vi "SDT_MeasureBlockToString.vi"(11 "MeasureInfo":T1={"mod_ser_no"="3F0024\u0000\u0000\u0000\u0000\u0000\u0000\u0000\u0000\u0000\u0000", "MeasureInfo_PartB"={"meas_mode"=13, "cfd_ll"=-29.411764, "cfd_lh"=5.019608, "cfd_zc"=12.850393, "cfd_hf"=5.0, "syn_zc"=-5.2913384, "syn_fd"=1, "syn_hf"=4.0, "tac_r"=5.0033574e-08, "tac_g"=3, "tac_of"=7.45098, "tac_ll"=5.098039, "tac_lh"=95.29412, "adc_re"=4096, "eal_de"=0, "ncx"=1, "ncy"=1, "page"=1, "col_t"=20.0, "rep_t"=20.0, "stopt"=0, "overfl"=78, "use_motor"=0, "steps"=1, "offset"=0.0, "dither"=128, "incr"=1, "mem_bank"=0, "mod_type1"=3722795091, "mod_type2"=0, "syn_th"=-50.980392, "dead_time_comp"=0, "polarity_l"=1, "polarity_f"=1, "polarity_p"=1, "linediv"=0, "accumulate"=0, "flbck_y"=1, "flbck_x"=1, "bord_u"=0, "bord_l"=0, "pix_time"=2e-07, "pix_clk"=1, "trigger"=16, "scan_x"=512, "scan_y"=512, "scan_rx"=1, "scan_ry"=1, "fifo_typ"=0, "epx_div"=1, "mod_type_code"=150, "mod_fpga_ver"=514, "overflow_corr_factor"=0.0, "adc_zoom"=0, "cycles"=1}, "MeasStopInfo"={"status"=824, "flags"=33199, "stop_time"=377.24805, "cur_step"=1, "cur_cycle"=1, "cur_page"=1, "min_sync_rate"=12634368.0, "min_cfd_rate"=1056.0, "min_tac_rate"=1056.0, "min_adc_rate"=70432.0, "max_sync_rate"=40678656.0, "max_cfd_rate"=769936.0, "max_tac_rate"=581984.0, "max_adc_rate"=565856.0, "reserved1"=0, "reserved2"=0.0}, "MeasFCSInfo"={"chan"=1, "fcs_decay_calc"=32, "mt_resol"=250, "cortime"=1.0, "calc_photons"=164220395, "fcs_points"=0, "end_time"=377.2369, "overruns"=0, "fcs_type"=32801, "cross_chan"=8, "mod"=0, "cross_mod"=0, "cross_mt_resol"=250}, "MeasureInfo_PartE"={"image_x"=512, "image_Y"=512, "image_rx"=1, "image_ry"=1, "xy_gain"=0, "dig_flags"=0, "adc_de"=0, "det_type"=0, "x_axis"=0}, "MeasHISTInfo"={"fida_time"=0.0, "filda_time"=0.0, "fida_points"=258, "filda_points"=511, "mcs_time"=0.0, "mcs_points"=512, "cross_calc_phot"=0, "mcsta_points"=0, "mcsta_flags"=0, "mcsta_tpp"=0, "calc_markers"=0, "fcs_calc_phot"=0, "reserved3"=0}, "HISTInfoExt"={"first_frame_time"=0.10108537, "frame_time"=1.4619007, "line_time"=0.002849475, "pixel_time"=4.4e-06, "scan_type"=0, "skip_2nd_line_clk"=0, "right_border"=0}, "MeasureInfo_PartF"={"sync_delay"=0.0, "sdel_ser_no"=0, "sdel_input"=0, "mosaic_ctrl"=0, "mosaic_x"=4, "mosaic_y"=4, "frames_per_el"=2, "chan_per_el"=1, "mosaic_cycles_done"=0, "mla_ser_no"=0, "DCC_in_use"=17}, "dcc_ser_no"="8A0043\u0000\u0000\u0000\u0000\u0000\u0000", "MeasureInfo_PartG"={"TiSaLas_status"=0, "TiSaLas_wav"=0, "AOM_status"=0, "AOM_power"=0}, "ddg_ser_no"="\u0000\u0000\u0000\u0000\u0000\u0000\u0000\u0000", "MeasureInfo"={"prior_ser_no"=0, "mosaic_x_hi"=0, "mosaic_y_hi"=0}} {"MeasFCSInfo"."fcs_decay_calc" format="%x"; "MeasStopInfo"."flags" format="x%x"; "MeasureInfo_PartB"."mod_type2" format="%016x"; "MeasureInfo_PartB"."mod_type1" format="%016x"}) -> (2 "length":i32, 3 "MeasureBlockString":string)   [LabVIEW 2017]
doc: "This VI is a SubVI to SDT_GenerateMeasureInfoBlock.vi. It formats the cluster MeasureInfo to a string ready to be written to file. \nParticular care is taken to format MeasureInfo's strings to the correct length. \n\ninfo@becker-hickl.com"
uses:
  SPC_Wrappers/SPC_Controls/MeasureInfo.ctl
  SPC_Wrappers/SPC_Controls/MeasureInfo_PartB.ctl
  SPC_Wrappers/SPC_Controls/MeasStopInfo.ctl
  SPC_Wrappers/SPC_Controls/MeasFCSInfo.ctl
  SPC_Wrappers/SPC_Controls/MeasureInfo_PartE.ctl
  SPC_Wrappers/SPC_Controls/MeasHISTInfo.ctl
  SPC_Wrappers/SPC_Controls/HISTInfoExt.ctl
  SPC_Wrappers/SPC_Controls/MeasureInfo_PartI.ctl
  SPC_Wrappers/SPC_Controls/MeasureInfo_PartK.ctl
  SPC_Wrappers/SPC_Controls/MeasureInfo_PartM.ctl
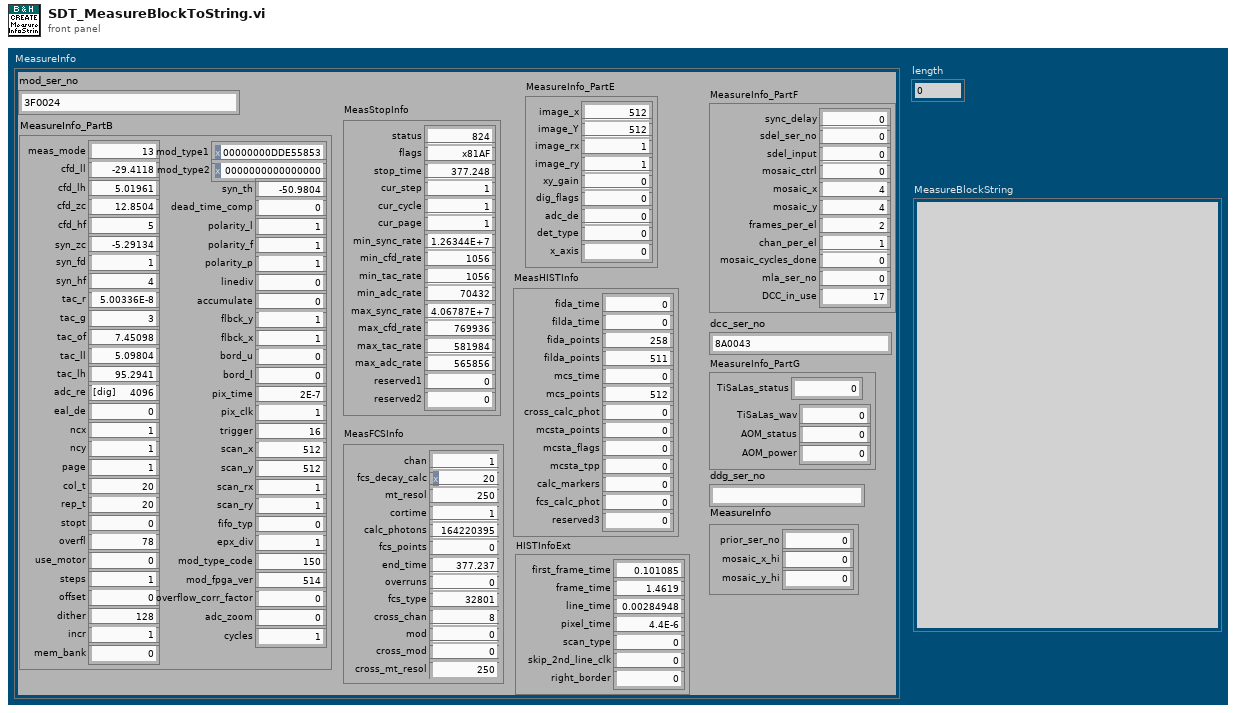
[diagram p1: front panel]
types:
  T1 = typedef "MeasureInfo.ctl" = cluster{"mod_ser_no":string, "MeasureInfo_PartB":T2, "MeasStopInfo":T3, "MeasFCSInfo":T4, "MeasureInfo_PartE":T5, "MeasHISTInfo":T6, "HISTInfoExt":T7, "MeasureInfo_PartF":T8, "dcc_ser_no":string, "MeasureInfo_PartG":T9, "ddg_ser_no":string, "MeasureInfo":T10}
  T2 = typedef "MeasureInfo_PartB.ctl" = cluster{"meas_mode":i16, "cfd_ll":sgl, "cfd_lh":sgl, "cfd_zc":sgl, "cfd_hf":sgl, "syn_zc":sgl, "syn_fd":i16, "syn_hf":sgl, "tac_r":sgl, "tac_g":i16, "tac_of":sgl, "tac_ll":sgl, "tac_lh":sgl, "adc_re":i16, "eal_de":i16, "ncx":i16, "ncy":i16, "page":u16, "col_t":sgl, "rep_t":sgl, "stopt":i16, "overfl":i8, "use_motor":i16, "steps":u16, "offset":sgl, "dither":i16, "incr":i16, "mem_bank":i16, "mod_type1":u64, "mod_type2":u64, "syn_th":sgl, "dead_time_comp":i16, "polarity_l":i16, "polarity_f":i16, "polarity_p":i16, "linediv":i16, "accumulate":i16, "flbck_y":i32, "flbck_x":i32, "bord_u":i32, "bord_l":i32, "pix_time":sgl, "pix_clk":i16, "trigger":i16, "scan_x":i32, "scan_y":i32, "scan_rx":i32, "scan_ry":i32, "fifo_typ":i16, "epx_div":i32, "mod_type_code":u16, "mod_fpga_ver":u16, "overflow_corr_factor":sgl, "adc_zoom":i32, "cycles":i32}
  T3 = typedef "MeasStopInfo.ctl" = cluster{"status":u16, "flags":u16, "stop_time":sgl, "cur_step":i32, "cur_cycle":i32, "cur_page":i32, "min_sync_rate":sgl, "min_cfd_rate":sgl, "min_tac_rate":sgl, "min_adc_rate":sgl, "max_sync_rate":sgl, "max_cfd_rate":sgl, "max_tac_rate":sgl, "max_adc_rate":sgl, "reserved1":i32, "reserved2":sgl}
  T4 = typedef "MeasFCSInfo.ctl" = cluster{"chan":u16, "fcs_decay_calc":u16, "mt_resol":u32, "cortime":sgl, "calc_photons":u32, "fcs_points":i32, "end_time":sgl, "overruns":u16, "fcs_type":u16, "cross_chan":u16, "mod":u16, "cross_mod":u16, "cross_mt_resol":u32}
  T5 = typedef "MeasureInfo_PartE.ctl" = cluster{"image_x":i32, "image_Y":i32, "image_rx":i32, "image_ry":i32, "xy_gain":i16, "dig_flags":i16, "adc_de":i16, "det_type":i16, "x_axis":i16}
  T6 = typedef "MeasHISTInfo.ctl" = cluster{"fida_time":sgl, "filda_time":sgl, "fida_points":i32, "filda_points":i32, "mcs_time":sgl, "mcs_points":i32, "cross_calc_phot":u32, "mcsta_points":u16, "mcsta_flags":u16, "mcsta_tpp":u32, "calc_markers":u32, "fcs_calc_phot":u32, "reserved3":u32}
  T7 = typedef "HISTInfoExt.ctl" = cluster{"first_frame_time":sgl, "frame_time":sgl, "line_time":sgl, "pixel_time":sgl, "scan_type":i16, "skip_2nd_line_clk":i16, "right_border":u32}
  T8 = typedef "MeasureInfo_PartI.ctl" = cluster{"sync_delay":sgl, "sdel_ser_no":u16, "sdel_input":i8, "mosaic_ctrl":i8, "mosaic_x":u8, "mosaic_y":u8, "frames_per_el":i16, "chan_per_el":i16, "mosaic_cycles_done":i32, "mla_ser_no":u16, "DCC_in_use":u8}
  T9 = typedef "MeasureInfo_PartK.ctl" = cluster{"TiSaLas_status":u16, "TiSaLas_wav":u16, "AOM_status":u8, "AOM_power":u8}
  T10 = typedef "MeasureInfo_PartM.ctl" = cluster{"prior_ser_no":i32, "mosaic_x_hi":u8, "mosaic_y_hi":u8}
  T11 = enum16{"big-endian, network order", "native, host order", "little-endian"}
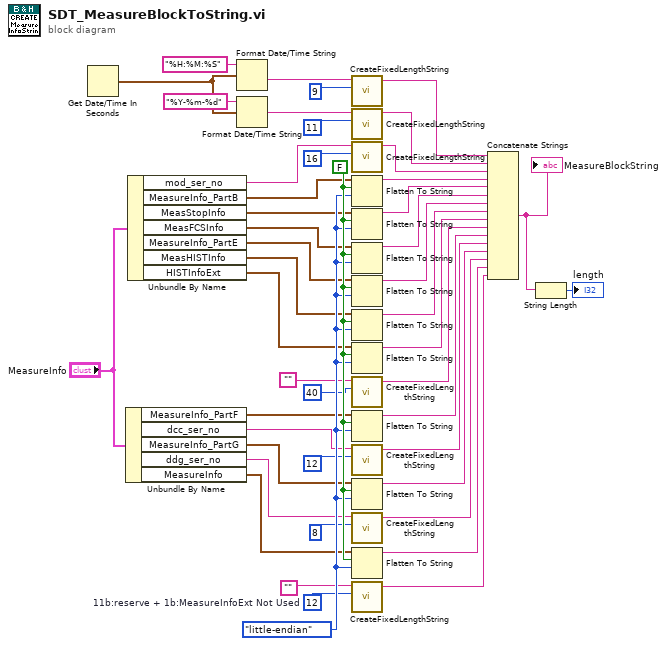
[diagram p0: block diagram]
diagram:
  w43 = T11."little-endian" ("byte order (0:big-endian, network order)")
  w44 = FALSE ("prepend array or string size? (T)")
  w8 = 12  # 11b:reserve + 1b:MeasureInfoExt Not Used
  n1 = Get Date/Time In Seconds() -> (seconds since 1Jan1904=w47:timestamp)
  n2 = Unbundle By Name("MeasureInfo") -> ("MeasureInfo_PartF"=w24:T8, "dcc_ser_no"=w12:string, "MeasureInfo_PartG"=w23:T9, "ddg_ser_no"=w10:string, "MeasureInfo"=w22:T10)
  n3 = Unbundle By Name("MeasureInfo") -> ("mod_ser_no"=w16:string, "MeasureInfo_PartB"=w31:T2, "MeasStopInfo"=w30:T3, "MeasFCSInfo"=w29:T4, "MeasureInfo_PartE"=w28:T5, "MeasHISTInfo"=w27:T6, "HISTInfoExt"=w26:T7)
  n4 = Format Date/Time String(time format string (%c)="%H:%M:%S", seconds (now)=w47) -> (date/time string=w21:string)  [unwired: 1 in]
  n5 = Format Date/Time String(time format string (%c)="%Y-%m-%d", seconds (now)=w47) -> (date/time string=w18:string)  [unwired: 1 in]
  n6 = call "CreateFixedLengthString.vi"("RequiredStringLength"=9 ("dimension size"), "StringIn"=w21) -> ("DLLString"=w20:string)  [unwired: 8 in, 1 out]
  n7 = call "CreateFixedLengthString.vi"("RequiredStringLength"=11 ("dimension size"), "StringIn"=w18) -> ("DLLString"=w1:string)  [unwired: 8 in, 1 out]
  n8 = call "CreateFixedLengthString.vi"("RequiredStringLength"=16 ("dimension size"), "StringIn"=w16) -> ("DLLString"=w2:string)  [unwired: 8 in, 1 out]
  n9 = Flatten To String(anything=w31, prepend array or string size? (T)=w44, byte order (0:big-endian, network order)=w43) -> (data string=w42:string)  [unwired: 1 in, 2 out]
  n10 = Flatten To String(anything=w30, prepend array or string size? (T)=w44, byte order (0:big-endian, network order)=w43) -> (data string=w41:string)  [unwired: 1 in, 2 out]
  n11 = Flatten To String(anything=w29, prepend array or string size? (T)=w44, byte order (0:big-endian, network order)=w43) -> (data string=w40:string)  [unwired: 1 in, 2 out]
  n12 = Flatten To String(anything=w28, prepend array or string size? (T)=w44, byte order (0:big-endian, network order)=w43) -> (data string=w39:string)  [unwired: 1 in, 2 out]
  n13 = Flatten To String(anything=w27, prepend array or string size? (T)=w44, byte order (0:big-endian, network order)=w43) -> (data string=w38:string)  [unwired: 1 in, 2 out]
  n14 = Flatten To String(anything=w26, prepend array or string size? (T)=w44, byte order (0:big-endian, network order)=w43) -> (data string=w37:string)  [unwired: 1 in, 2 out]
  n15 = call "CreateFixedLengthString.vi"("RequiredStringLength"=40 ("dimension size"), "StringIn"="") -> ("DLLString"=w3:string)  [unwired: 8 in, 1 out]
  n16 = Flatten To String(anything=w24, prepend array or string size? (T)=w44, byte order (0:big-endian, network order)=w43) -> (data string=w36:string)  [unwired: 1 in, 2 out]
  n17 = call "CreateFixedLengthString.vi"("RequiredStringLength"=12 ("dimension size"), "StringIn"=w12) -> ("DLLString"=w4:string)  [unwired: 8 in, 1 out]
  n18 = Flatten To String(anything=w23, prepend array or string size? (T)=w44, byte order (0:big-endian, network order)=w43) -> (data string=w35:string)  [unwired: 1 in, 2 out]
  n19 = call "CreateFixedLengthString.vi"("RequiredStringLength"=8 ("dimension size"), "StringIn"=w10) -> ("DLLString"=w5:string)  [unwired: 8 in, 1 out]
  n20 = Flatten To String(anything=w22, prepend array or string size? (T)=w44, byte order (0:big-endian, network order)=w43) -> (data string=w34:string)  [unwired: 1 in, 2 out]
  n21 = call "CreateFixedLengthString.vi"("RequiredStringLength"=w8, "StringIn"="") -> ("DLLString"=w6:string)  [unwired: 8 in, 1 out]
  n22 = Concatenate Strings(w20, w1, w2, w42, w41, w40, w39, w38, w37, w3, w36, w4, w35, w5, w34, w6) -> (w33:string)
  "MeasureBlockString" <- w33
  n23 = String Length(string=w33) -> (length=→"length":i32)
